vi "LS Acquisition Main (FPGA).vi"() -> ()   [LabVIEW 2019]
uses:
  <vilib>/rvi/Emulation/niFpgaGetClockAttributes.vi
  <vilib>/rvi/Emulation/niFpgaSctlEmulationGetInTimedLoop.vi
  <vilib>/rvi/Emulation/niFpgaEmulationReportErrorSimple.vi
  <vilib>/rvi/Emulation/niFpgaProcessEmulError.vi
  <vilib>/rvi/eio/common/nirviEmuTemplateMethod_errors.vi
  <vilib>/rvi/Emulation/niFpgaCriticalErrorInLSC.vi
  <vilib>/rvi/DataTransferAndStorage/Container/Common/niFpgaContainerExecOnDevCompGetState.vi
  <vilib>/rvi/Emulation/niFpgaEmulationIsFPGAContextNoSignature.vi
  <vilib>/rvi/errors/niFpgaSetErrorForExecOnDevCompSimple.vi
  <vilib>/rvi/eio/common/nirviEmuReportErrorAndStop.vi
  <vilib>/rvi/DataTransferAndStorage/Container/Common/niFpgaContainerGetUniqueNameForEmu.vi
  <vilib>/rvi/FIFO/Fifo_Resource/nirvififoEmulationSetSize.vi
  <vilib>/rvi/FIFO/Fifo_Resource/nirviFifoEmulationQueueMgr.vi
  <instcachedir>/0/nirviFifoEmulationQueueMgr_E5CAEC123FF24DC58D834DCA3CDAA9B5.lvgen/nirviFifoEmulationQueueMgr_E5CAEC123FF24DC58D834DCA3CDAA9B5_002.vi
  <vilib>/rvi/FIFO/Fifo_Resource/nirvififoEmulationDetermineInputValidOut.vi
  <vilib>/rvi/FIFO/Fifo_Resource/nirvififoEmulationCreateLock.vi
  <vilib>/rvi/FIFO/Fifo_Resource/nirvififoEmulationObtainLock.vi
  <vilib>/rvi/FIFO/Fifo_Resource/nirvififoEmulationReleaseLock.vi
  <vilib>/rvi/occurrence/nirviWaitOnOccurrenceBase.vi
  <vilib>/rvi/errors/nirviReportUnexpectedCaseInternalError.vi
  <vilib>/rvi/errors/nirviReportUnexpectedCaseInternalError (U32).vi
  <vilib>/Utility/error.llb/Clear Errors.vi
  <vilib>/rvi/interface/RandomDataEmulation/niFpgaRandomDataHandleErrors.vi
  <vilib>/eio/EIONode/EIONode.xnode
  <vilib>/rvi/FXPMathLib/FxpAdd/XNode/nifxpmath_Add.xnode
  <vilib>/rvi/DataTransferAndStorage/Container/XNode/niFpgaContainer.xnode
  <vilib>/rvi/FIFO/Fifo_Resource/niFpgaFifoEmulationRefIn.vi
  <vilib>/rvi/FXPMathLib/sim/FxpSim.dll
panel:
  in  "AI Set Time(uSec)":u32=80
  in  "B2offset":fxp<+/-,24,5>
  in  "B1offset":fxp<+/-,24,5>
  out "Anomaly Resamples":fxp<+/-,28,17>[](array[numeric])
  out "Bank2Active":bool
  out "Bank1Active":bool
  out "Bank2On":bool
  out "Bank1On":bool
  in  "Enable Readings":bool[](array[boolean])=[FALSE, FALSE, FALSE, FALSE, FALSE, FALSE, FALSE, FALSE, FALSE, FALSE, FALSE, FALSE]
  in  "Opens Resets":bool[](array[boolean])=[FALSE, FALSE, FALSE, FALSE, FALSE, FALSE, FALSE, FALSE, FALSE, FALSE]
  in  "Enable Opens":bool[](array[boolean])=[FALSE, FALSE, FALSE, FALSE, FALSE, FALSE, FALSE, FALSE, FALSE, FALSE]
  out "Opens Detected":u16[](array[numeric])
  out "Opens Loop Time (usec)":u32=1000
  in  "Bank2(Pulse/Const)":bool
  in  "Bank2Const(On/Off)":bool
  out "Cycle Starts":bool[](array[boolean])
  out "Cycles":u32[](array[numeric])
  in  "Bank1Const(On/Off)":bool
  in  "Bank1(Pulse/Const)":bool
  in  "PWM Period (Ticks)":u32=4000000
  in  "Duty (Ticks)":i32=2000000
  in  "Invert PWM?":bool=TRUE
  in  "Cycle Resets":bool[](array[boolean])=[FALSE, FALSE, FALSE, FALSE, FALSE, FALSE, FALSE, FALSE, FALSE, FALSE]
  in  "Points to Avg":i32=20
  in  "Enable Cycles":bool[](array[boolean])=[FALSE, FALSE, FALSE, FALSE, FALSE, FALSE, FALSE, FALSE, FALSE, FALSE]
  out "Total Cycles":u32[](array[numeric])
  in  "Cycle Threshold":fxp<+/-,28,17>=1.2001953125
  out "Analog Inputs":fxp<+/-,28,17>[](array[numeric])
  out "AI Loop Time (usec)":u32=70
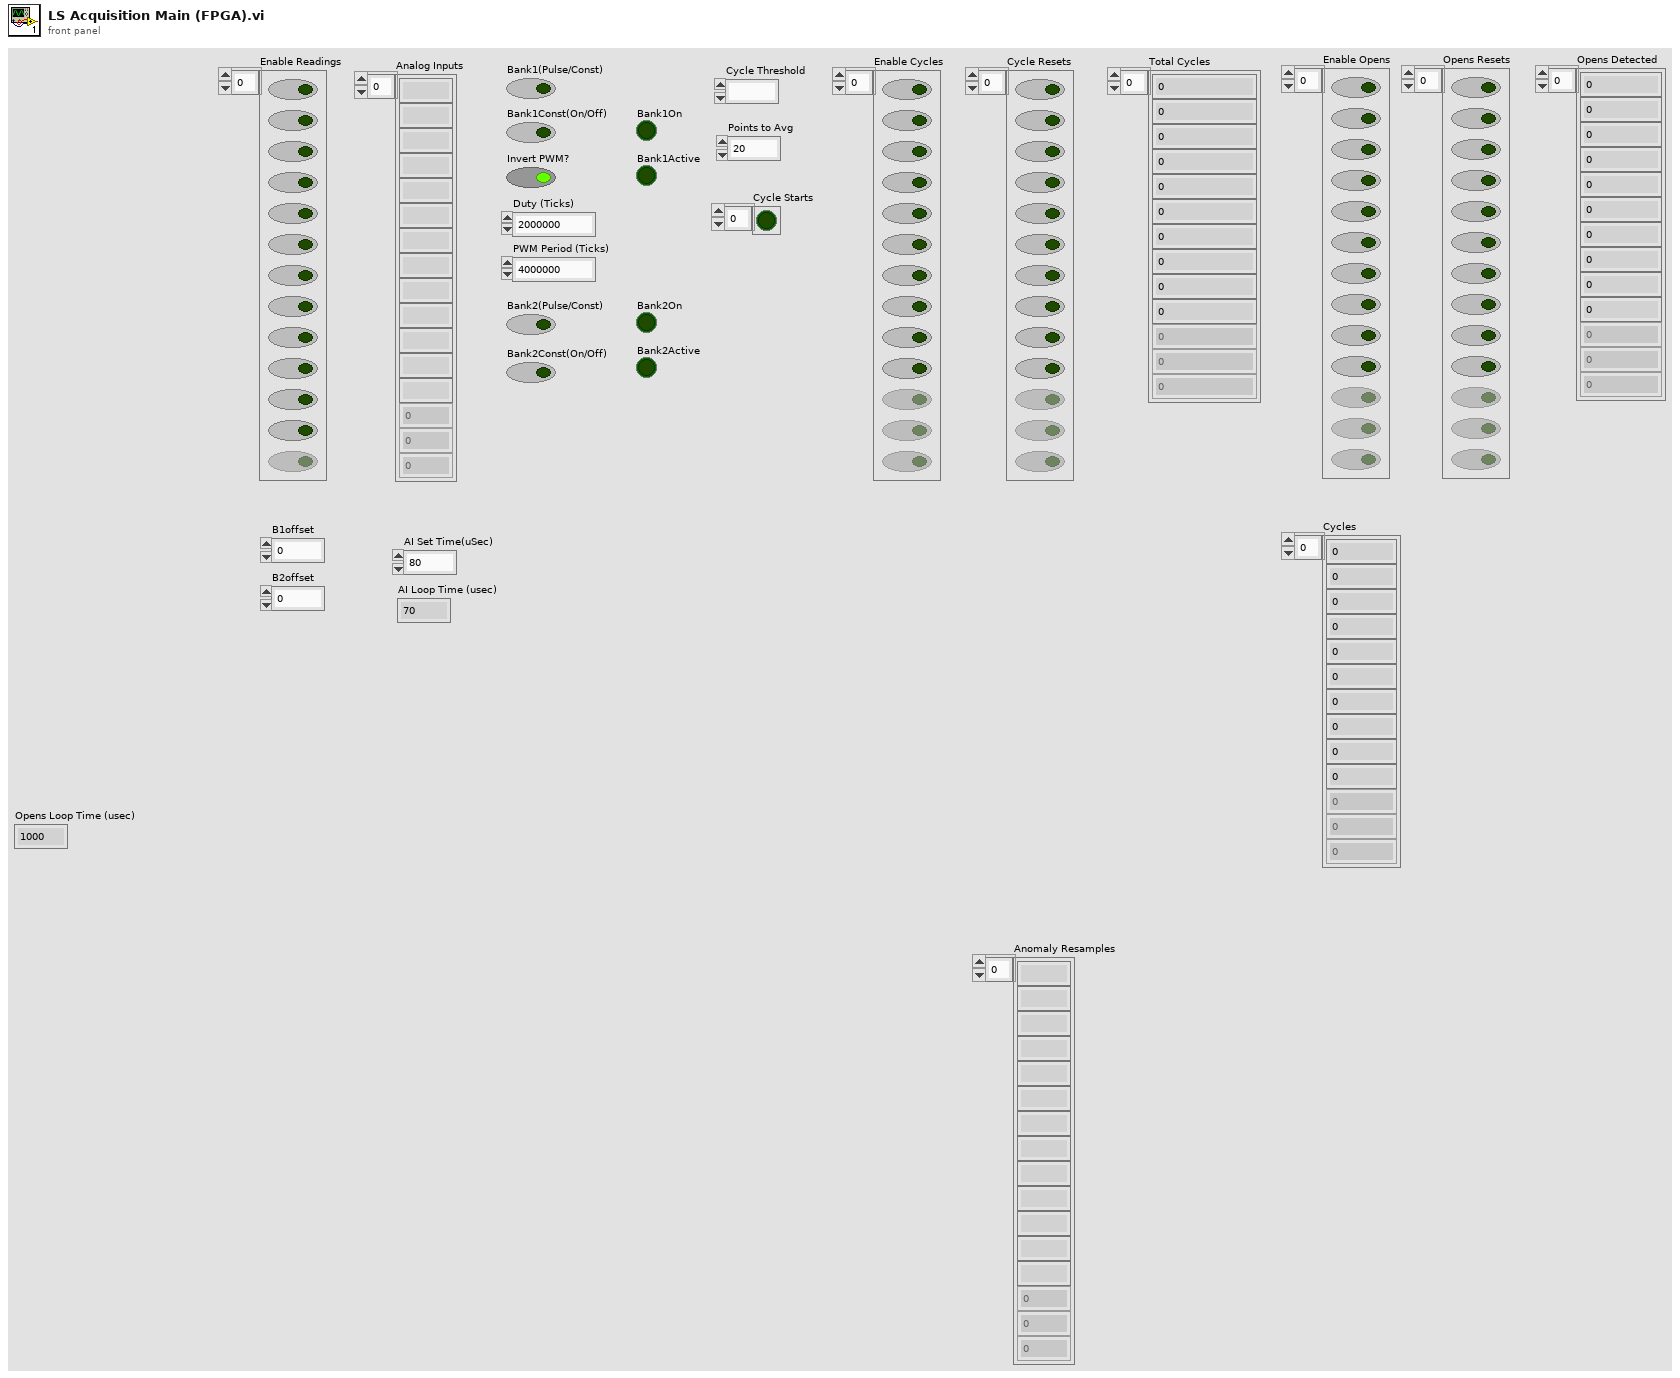
[diagram p1: front panel]
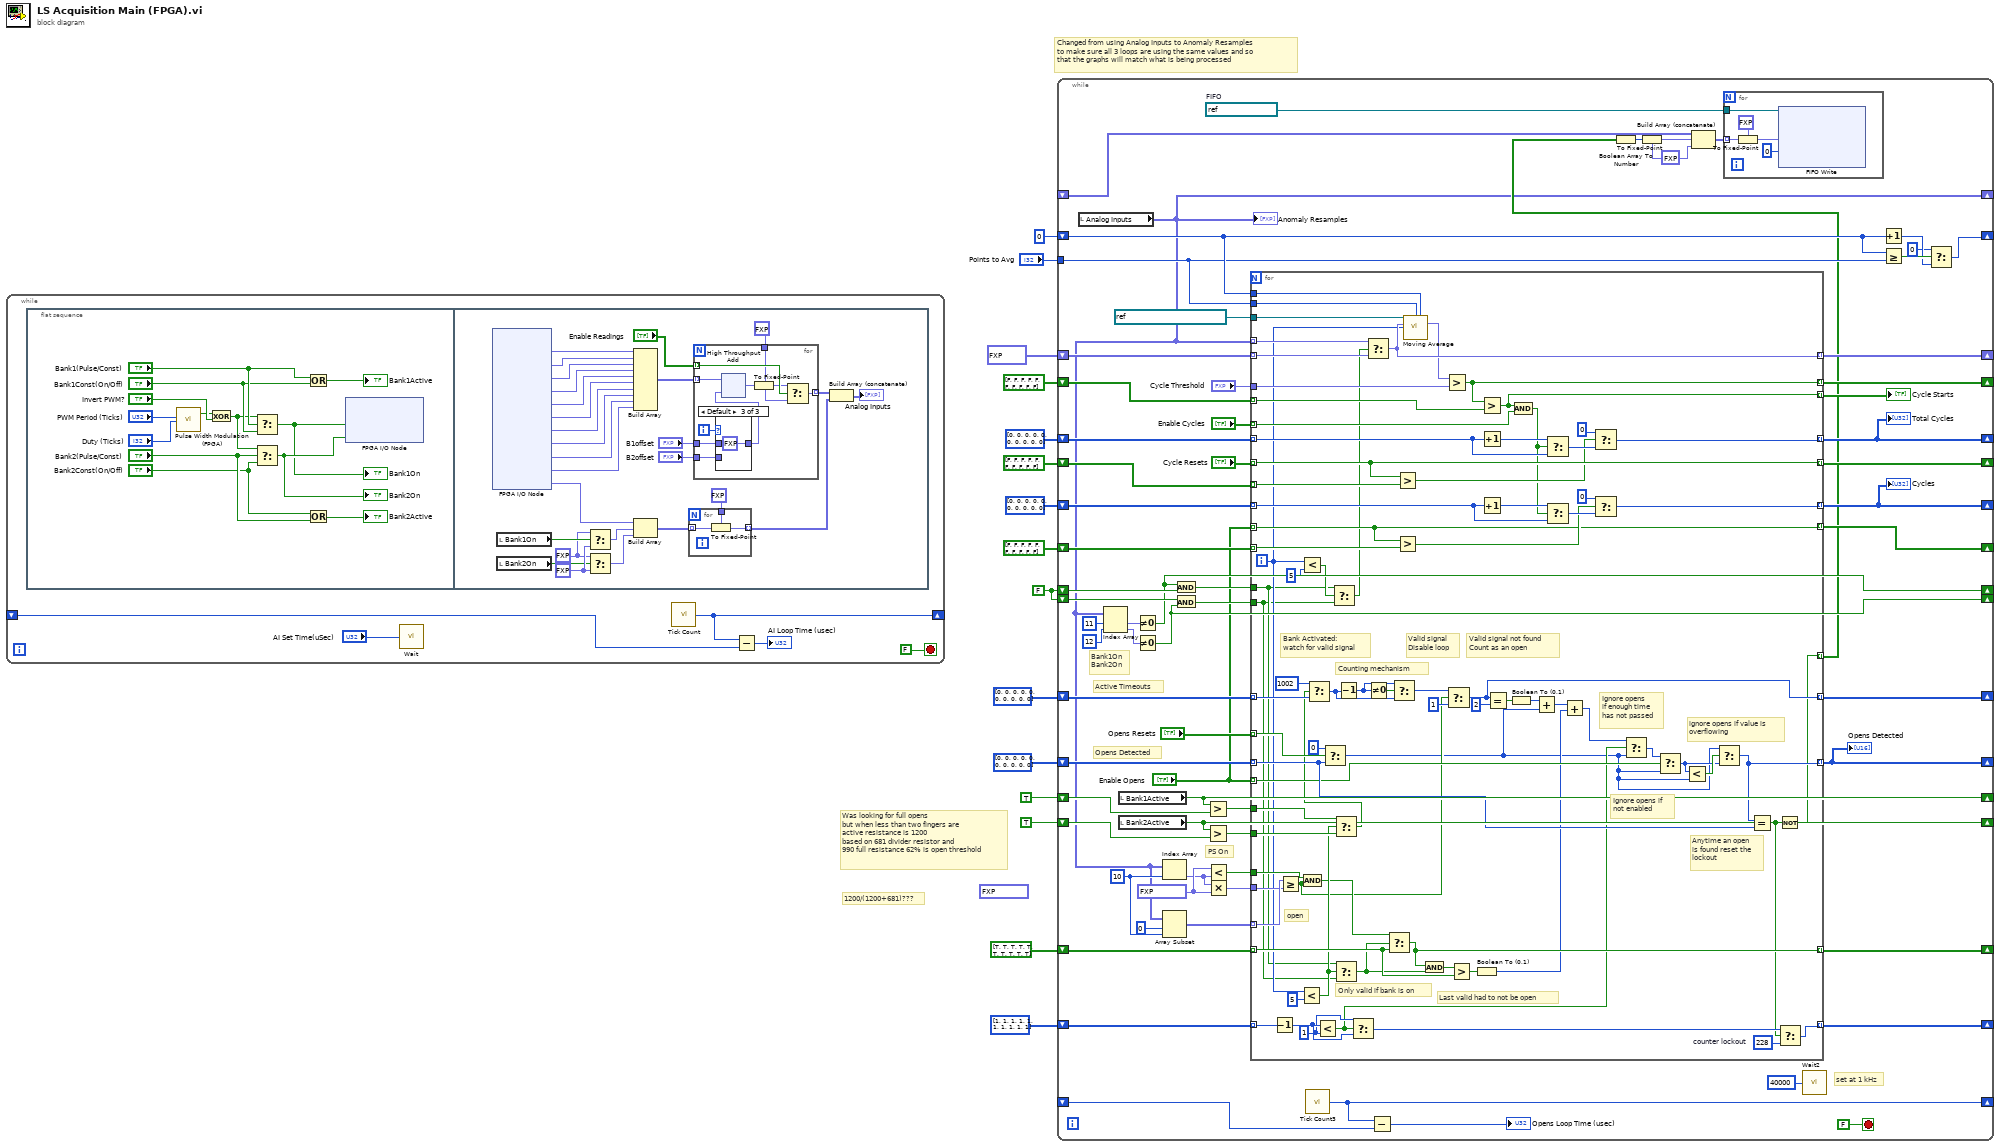
[diagram p0: block diagram]
diagram:
  (unwired) fxp<+,8,0> 0.94921875
  w7 = FALSE
  # "1200/(1200+681)???"
  # "Was looking for full opens\nbut when less than two fingers are\nactive resistance is 1200\nbased on 681 divider resistor and\n990 full resistance 62% is open threshold"
  # "Changed from using Analog Inputs to Anomaly Resamples\nto make sure all 3 loops are using the same values and so\nthat the graphs will match what is being processed"
  n1 = while {
    shift-right: [w19] -> _
    shift-left: _ -> [w18]
    stop <- FALSE stop-if-true
    n2 = flat-sequence {
      frame #0 {
        n3 = call "Pulse Width Modulation (FPGA).vi"("PWM Period (Ticks)"="PWM Period (Ticks)", "PWM Duty Cycle (Ticks)"="Duty (Ticks)") -> ("PWM DO"=w23:bool)  [unwired: 14 in, 3 out]
        n4 = Exclusive Or(1:"Invert PWM?", 2:w23) -> (0:w25:bool)
        n5 = Select(t=w25, s="Bank1(Pulse/Const)", f="Bank1Const(On/Off)") -> (s? t:f=w26:bool)
        "Bank1On" <- w26
        n6 = Select(t=w25, s="Bank2(Pulse/Const)", f="Bank2Const(On/Off)") -> (s? t:f=w27:bool)
        "Bank2On" <- w27
        n7 = Or(x="Bank1(Pulse/Const)", y="Bank1Const(On/Off)") -> (x .or. y?=→"Bank1Active":bool)
        n8 = Or(x="Bank2Const(On/Off)", y="Bank2(Pulse/Const)") -> (x .or. y?=→"Bank2Active":bool)
        n9 = xnode "FPGA I/O Node"("RMC/DIO0"=w26, "RMC/DIO1"=w27) -> ()  [unwired: 3 in, 3 out]
      }
      frame #1 {
        w38 = fxp<+/-,24,5> 1.0 ("AI13")
        w41 = fxp<+/-,24,5> 0.0 ("AI13")
        n10 = xnode "FPGA I/O Node"() -> ("AI0"=w60:fxp<+/-,24,5>, "AI1"=w59:fxp<+/-,24,5>, "AI2"=w58:fxp<+/-,24,5>, "AI3"=w57:fxp<+/-,24,5>, "AI4"=w56:fxp<+/-,24,5>, "AI6"=w55:fxp<+/-,24,5>, "AI7"=w54:fxp<+/-,24,5>, "AI8"=w53:fxp<+/-,24,5>, "AI9"=w52:fxp<+/-,24,5>, "AI10"=w51:fxp<+/-,24,5>, "AI12"=w48:fxp<+/-,24,5>)  [unwired: 11 in, 11 out]
        n11 = local read "Bank1On"() -> (w40:bool)
        n12 = local read "Bank2On"() -> (w39:bool)
        n13 = Select(t=w38, s=w40, f=w41) -> (s? t:f=w37:fxp<+/-,24,5>)
        n14 = Select(t=w38, s=w39, f=w41) -> (s? t:f=w36:fxp<+/-,24,5>)
        n15 = Build Array(w60, w59, w58, w57, w56, w55, w54, w53, w52, w51) -> (w50:fxp<+/-,24,5>[])
        n16 = Build Array(w48, w37, w36) -> (w46:fxp<+/-,24,5>[])
        n17 = for {
          tunnel: w46 -> [w63] mode=indexing
          tunnel: fxp<+/-,28,17> 0.0 ("AI0") -> [w62]
          tunnel: [w61] -> w45 mode=indexing
          n18 = To Fixed-Point(fixed-point type=w62, number=w63) -> (fixed-point=w61:fxp<+/-,28,17>)
        }
        n19 = for {
          tunnel: w50 -> [w66] mode=indexing
          tunnel: fxp<+/-,28,17> 0.0 ("AI0") -> [w71]
          tunnel: [w70] -> w44 mode=indexing
          tunnel: "Enable Readings" -> [w73] mode=indexing
          tunnel: "B1offset" -> [w68]
          tunnel: "B2offset" -> [w67]
          i -> [w69]
          n20 = case shown="Default" w69 {
            tunnel: w68 -> [w74 _ _]
            tunnel: w67 -> [_ w75 _]
            tunnel: [w74 w75 fxp<+/-,24,5> 0.0 ("B2offset")] -> w65
            frame 0..4 {
            }
            frame 5..9 {
            }
            frame Default {
            }
          }
          n21 = xnode ("High Throughput Add")("x"=w66, "y"=w65) -> ("x+y"=w64:fxp<+/-,25,6>)
          n22 = To Fixed-Point(fixed-point type=w71, number=w64) -> (fixed-point=w72:fxp<+/-,28,17>)
          n23 = Select(t=w72, s=w73, f=w71) -> (s? t:f=w70:fxp<+/-,28,17>)
        }
        n24 = Build Array (concatenate)(w44, w45) -> (→"Analog Inputs":fxp<+/-,28,17>[])
      }
    }
    n25 = call "Wait"("Count(uSec)"="AI Set Time(uSec)") -> ()  [unwired: 1 out]
    n26 = call "Tick Count"() -> ("Tick Count(uSec)"=w19:u32)
    n27 = Subtract(x=w19, y=w18) -> (x-y=→"AI Loop Time (usec)":u32)
  }
  n28 = while {
    shift-right: [w143] -> _
    shift-left: _ -> [w142]
    shift-right: [w108] -> _
    shift-right: [w109] -> _
    shift-left: w7 -> [w138]
    shift-left: w7 -> [w139]
    tunnel: "Points to Avg" -> [w115]
    shift-right: [w134] -> _
    shift-left: 0 ("Moving Point Index") -> [w116]
    shift-right: [w117] -> _
    shift-left: fxp<+/-,28,17>[] [0.0, 0.0, 0.0, 0.0, 0.0, 0.0, 0.0, 0.0, 0.0, 0.0] ("Analog Inputs") -> [w119]
    shift-right: [w120] -> _
    shift-left: bool[] [FALSE, FALSE, FALSE, FALSE, FALSE, FALSE, FALSE, FALSE, FALSE, FALSE] -> [w122]
    shift-right: [w125] -> _
    shift-left: u32[] [0, 0, 0, 0, 0, 0, 0, 0, 0, 0] -> [w126]
    shift-right: [w127] -> _
    shift-left: bool[] [FALSE, FALSE, FALSE, FALSE, FALSE, FALSE, FALSE, FALSE, FALSE, FALSE] -> [w129]
    shift-right: [w131] -> _
    shift-left: u32[] [0, 0, 0, 0, 0, 0, 0, 0, 0, 0] -> [w132]
    shift-right: [w130] -> _
    shift-left: bool[] [FALSE, FALSE, FALSE, FALSE, FALSE, FALSE, FALSE, FALSE, FALSE, FALSE] -> [w133]
    shift-right: [w77] -> _
    shift-left: _ -> [w103]
    shift-right: [w96] -> _
    shift-left: u16[] [0, 0, 0, 0, 0, 0, 0, 0, 0, 0] -> [w100]
    shift-right: [w79] -> _
    shift-left: u8[] [0, 0, 0, 0, 0, 0, 0, 0, 0, 0] -> [w99]
    shift-right: [w85] -> _
    shift-left: TRUE ("Bank1Active") -> [w89]
    shift-right: [w84] -> _
    shift-left: TRUE ("Bank2Active") -> [w88]
    shift-right: [w95] -> _
    shift-left: bool[] [TRUE, TRUE, TRUE, TRUE, TRUE, TRUE, TRUE, TRUE, TRUE, TRUE] -> [w98]
    shift-right: [w94] -> _
    shift-left: u16[] [1, 1, 1, 1, 1, 1, 1, 1, 1, 1] -> [w97]
    stop <- FALSE stop-if-true
    w92 = fxp<+,8,0> 0.62890625
    w82 = 10 ("length")
    w104 = refnum<k21> "Analog Data"  # FIFO
    w106 = fxp<+/-,28,17> -15.0 ("AI0")
    # "PS On"
    # "Opens Detected"
    # "Active Timeouts"
    # "Bank1On\nBank2On"
    # "set at 1 kHz"
    n29 = local read "Analog Inputs"() -> (w77:fxp<+/-,28,17>[])
    "Anomaly Resamples" <- w77
    n30 = Index Array(array=w77, index #1=11 ("index"), index #2=12 ("index")) -> (element #1=w111:fxp<+/-,28,17>, element #2=w110:fxp<+/-,28,17>)
    n31 = local read "Bank1Active"() -> (w85:bool)
    n32 = local read "Bank2Active"() -> (w84:bool)
    n33 = Not Equal To 0?(x=w111) -> (x != 0?=w108:bool)
    n34 = Not Equal To 0?(x=w110) -> (x != 0?=w109:bool)
    n35 = Index Array(array=w77, index=w82) -> (element=w91:fxp<+/-,28,17>)
    n36 = Array Subset(array=w77, index=0, length=w82) -> (w83:fxp<+/-,28,17>[])
    n37 = And(x=w108, y=w139) -> (x .and. y?=w141:bool)
    n38 = And(x=w138, y=w109) -> (x .and. y?=w140:bool)
    n39 = Greater?(x=w85, y=w89) -> (0:w87:bool)
    n40 = Greater?(x=w84, y=w88) -> (0:w86:bool)
    n41 = Less?(x=w92, y=w91) -> (x < y?=w81:bool)
    n42 = Multiply(x=w91, y=w92) -> (x*y=w80:fxp<+/-,36,17>)
    n43 = for {
      tunnel: w141 -> [w154]
      tunnel: w140 -> [w153]
      tunnel: w133 -> [w231] mode=indexing
      tunnel: "Enable Opens" -> [w224] mode=indexing
      tunnel: w132 -> [w227] mode=indexing
      tunnel: [w226] -> w131 mode=indexing
      tunnel: [w224] -> w130 mode=indexing
      tunnel: w129 -> [w223] mode=indexing
      tunnel: "Cycle Resets" -> [w222] mode=indexing
      tunnel: [w222] -> w127 mode=indexing
      tunnel: w126 -> [w217] mode=indexing
      tunnel: [w216] -> w125 mode=indexing
      tunnel: "Enable Cycles" -> [w215] mode=indexing
      tunnel: "Cycle Threshold" -> [w212]
      tunnel: w122 -> [w213] mode=indexing
      tunnel: [w204] -> w121 mode=indexing
      tunnel: [w211] -> w120 mode=indexing
      tunnel: w119 -> [w210] mode=indexing
      tunnel: w77 -> [w201] mode=indexing
      tunnel: refnum<k21> "Running Avg Memory" ("Memory") -> [w209]
      tunnel: [w208] -> w117 mode=indexing
      tunnel: w116 -> [w207]
      tunnel: w115 -> [w206]
      tunnel: [w151] -> w102 mode=indexing
      tunnel: w100 -> [w200] mode=indexing
      tunnel: w99 -> [w199] mode=indexing
      tunnel: w98 -> [w198] mode=indexing
      tunnel: w97 -> [w197] mode=indexing
      tunnel: [w196] -> w96 mode=indexing
      tunnel: [w195] -> w95 mode=indexing
      tunnel: [w194] -> w94 mode=indexing
      tunnel: [w193] -> w79 mode=indexing
      tunnel: "Opens Resets" -> [w192] mode=indexing
      tunnel: "Enable Opens" -> [w191] mode=indexing
      tunnel: w87 -> [w190]
      tunnel: w86 -> [w189]
      tunnel: w83 -> [w188] mode=indexing
      tunnel: w81 -> [w187]
      tunnel: w80 -> [w186]
      i -> [w155]
      w160 = u16 228  # counter lockout
      w162 = u16 1 ("y")
      # "Ignore opens if\nnot enabled"
      # "Ignore opens\nif enough time\nhas not passed"
      # "Anytime an open\nis found reset the\nlockout"
      # "ignore opens if value is\noverflowing"
      # "Last valid had to not be open"
      # "Only valid if bank is on"
      # "open"
      # "Valid signal not found\nCount as an open"
      # "Valid signal\nDisable loop"
      # "Counting mechanism"
      # "Bank Activated:\nwatch for valid signal"
      n44 = Decrement(x=w197) -> (x-1=w163:u16)
      n45 = Greater Or Equal?(x=w188, y=w186) -> (x >= y?=w167:bool)
      n46 = Less?(x=w155, y=5) -> (x < y?=w184:bool)
      n47 = Less?(x=w155, y=5) -> (x < y?=w203:bool)
      n48 = And(x=w187, y=w167) -> (x .and. y?=w171:bool)
      n49 = Less?(x=w163, y=w162) -> (x < y?=w157:bool)
      n50 = Select(t=u16 0, s=w192, f=w199) -> (s? t:f=w156:u16)
      n51 = Select(t=w154, s=w203, f=w153) -> (s? t:f=w202:bool)
      n52 = Select(t=w190, s=w184, f=w189) -> (s? t:f=w172:bool)
      n53 = Select(t=u16 1002, s=w172, f=w200) -> (s? t:f=w173:u16)
      n54 = Select(t=w154, s=w184, f=w153) -> (s? t:f=w170:bool)
      n55 = Decrement(x=w173) -> (x-1=w177:u16)
      n56 = Select(t=w162, s=w157, f=w163) -> (s? t:f=w161:u16)
      n57 = Select(t=w201, s=w202, f=w210) -> (s? t:f=w208:fxp<+/-,28,17>)
      n58 = Not Equal To 0?(x=w177) -> (x != 0?=w176:bool)
      n59 = Select(t=w171, s=w170, f=w198) -> (s? t:f=w195:bool)
      n60 = Select(t=w177, s=w176, f=w173) -> (s? t:f=w178:u16)
      n61 = Greater?(x=w222, y=w223) -> (0:w218:bool)
      n62 = Greater?(x=w224, y=w231) -> (0:w225:bool)
      n63 = call "Moving Average.vi"("Memory In"=w209, "N (# of Ave Pts 127 max)"=w206, "Moving Point Index"=w207, "Data IN"=w208, "Channel#"=w155) -> ("Averaged Data"=w205:fxp<+/-,28,17>)  [unwired: 10 in]
      n64 = And(x=w195, y=w170) -> (x .and. y?=w166:bool)
      n65 = Greater?(x=w205, y=w212) -> (0:w211:bool)
      n66 = Select(t=w178, s=w167, f=u16 1) -> (s? t:f=w196:u16)
      n67 = Greater?(x=w166, y=w198) -> (0:w169:bool)
      n68 = Boolean To (0,1)(Boolean=w169) -> (0, 1=w168:i16)
      n69 = Greater?(x=w211, y=w213) -> (0:w204:bool)
      n70 = Increment(x=w217) -> (x+1=w219:u32)
      n71 = Increment(x=w227) -> (x+1=w230:u32)
      n72 = Equal?(x=w196, y=u16 2) -> (x = y?=w180:bool)
      n73 = Boolean To (0,1)(Boolean=w180) -> (0, 1=w181:i16)
      n74 = And(x=w204, y=w215) -> (x .and. y?=w214:bool)
      n75 = Add(x=w181, y=w156) -> (x+y=w182:u16)
      n76 = Select(t=w219, s=w214, f=w217) -> (s? t:f=w220:u32)
      n77 = Select(t=w230, s=w214, f=w227) -> (s? t:f=w229:u32)
      n78 = Add(x=w182, y=w168) -> (x+y=w158:u16)
      n79 = Select(t=u32 0, s=w218, f=w220) -> (s? t:f=w216:u32)
      n80 = Select(t=u32 0, s=w225, f=w229) -> (s? t:f=w226:u32)
      n81 = Select(t=w158, s=w157, f=w156) -> (s? t:f=w159:u16)
      n82 = Select(t=w159, s=w191, f=w156) -> (s? t:f=w164:u16)
      n83 = Less?(x=w164, y=w156) -> (x < y?=w165:bool)
      n84 = Select(t=w156, s=w165, f=w164) -> (s? t:f=w193:u16)
      n85 = Equal?(x=w193, y=w199) -> (x = y?=w152:bool)
      n86 = Not(x=w152) -> (.not. x?=w151:bool)
      n87 = Select(t=w161, s=w152, f=w160) -> (s? t:f=w194:u16)
    }
    "Total Cycles" <- w125
    "Cycles" <- w131
    "Cycle Starts" <- w121
    "Opens Detected" <- w79
    n88 = call "Tick Count3"() -> ("Tick Count(uSec)"=w143:u32)
    n89 = Subtract(x=w143, y=w142) -> (x-y=→"Opens Loop Time (usec)":u32)
    n90 = Boolean Array To Number(Boolean array=w102) -> (number=w107:u16)
    n91 = To Fixed-Point(fixed-point type=w106, number=w107) -> (fixed-point=w105:fxp<+/-,28,17>)
    n92 = Build Array (concatenate)(w103, w105, w106) -> (w114:fxp<+/-,28,17>[])
    n93 = for {
      tunnel: w104 -> [w150]
      tunnel: w114 -> [w149] mode=indexing
      n94 = To Fixed-Point(fixed-point type=fxp<+/-,22,11> 0.0 ("AI0"), number=w149) -> (fixed-point=w148:fxp<+/-,22,11>)
      n95 = xnode ("FIFO Write")("Element"=w148, "Timeout"=0, "FIFO In"=w150) -> ()  [unwired: 2 out]
    }
    n96 = call "Wait2"("Count(Ticks)"=u32 40000 ("Count(mSec)")) -> ()  [unwired: 1 out]
    n97 = Increment(x=w116) -> (x+1=w136:i32)
    n98 = Greater Or Equal?(x=w116, y=w115) -> (x >= y?=w137:bool)
    n99 = Select(t=0, s=w137, f=w136) -> (s? t:f=w134:i32)
  }
